vi "IsFPSSmaller.vi"(8 "error constant":errorcluster, 10 "Frame Rate":dbl, 11 "Max FrameRate":dbl) -> (0 "error out":errorcluster)   [LabVIEW 2023]
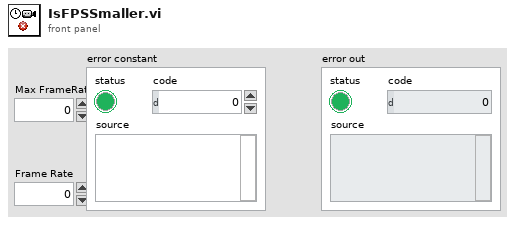
[diagram p1: front panel]
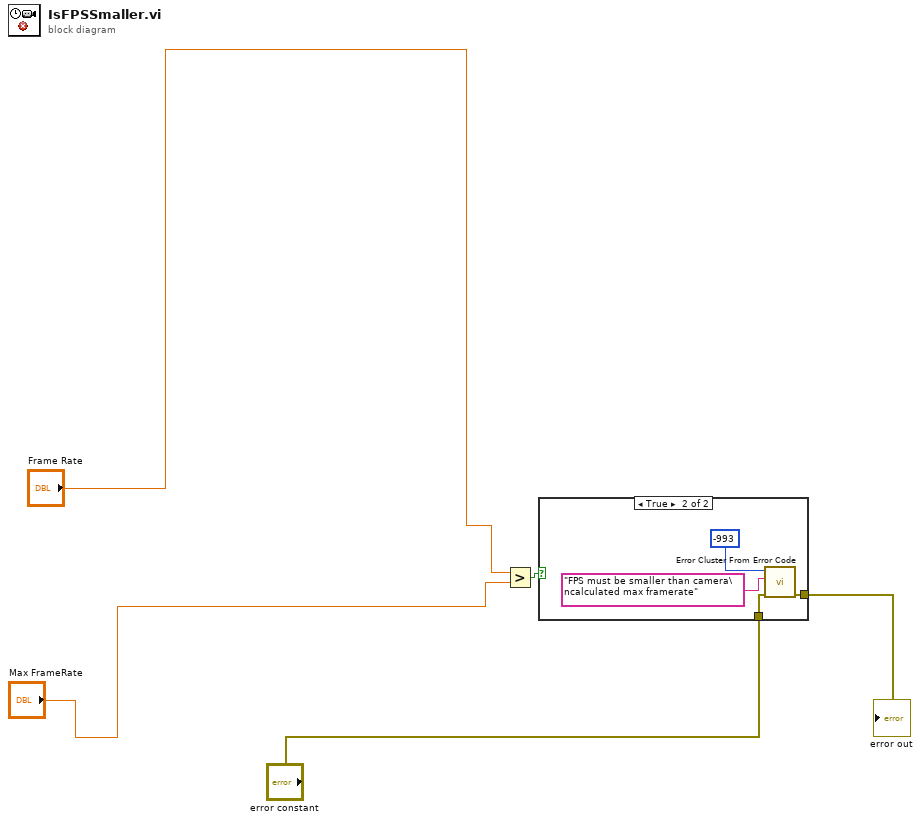
[diagram p0: block diagram]
diagram:
  n1 = Greater?(x="Frame Rate", y="Max FrameRate") -> (0:w5:bool)
  n2 = case shown="True" w5 {
    tunnel: "error constant" -> [w6 w8]
    tunnel: [w6 w7] -> w2
    frame False {
    }
    frame True {
      n3 = call <vilib>:"Error Cluster From Error Code.vi"("error in (no error)"=w8, "error message (\"\")"="FPS must be smaller than camera\ncalculated max framerate" ("error message (\"\")"), "error code (0)"=-993) -> ("error out"=w7:errorcluster)  [unwired: 6 in]
    }
  }
  "error out" <- w2
